vi "Dialog_Pause.vi"(11 "Wait (s)":dbl) -> ()   [LabVIEW 2012]
panel:
  in  "Cancel Button":bool
  out "Gauge":dbl(knob) scale=0.0..3.0
  out "Slide":dbl(slide) scale=0.0..3.0
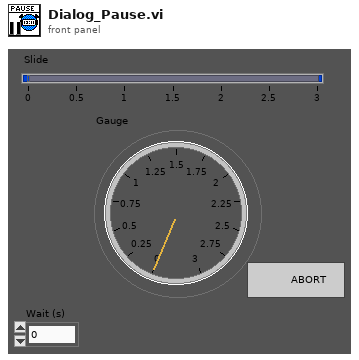
[diagram p1: front panel]
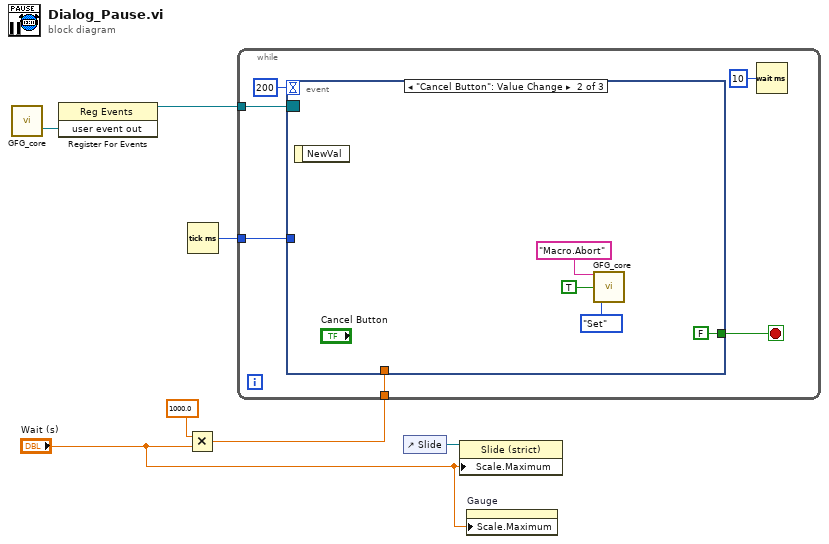
[diagram p0: block diagram]
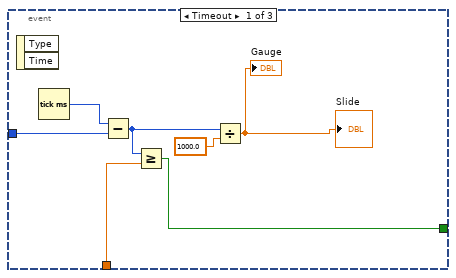
[diagram p2: hidden frame]
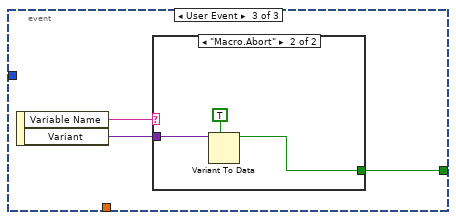
[diagram p3: hidden frame]
diagram:
  n1 = call "GFG_core.vi"() -> ("user event out"=w2:refnum<user-event>)  [unwired: 13 in, 6 out]
  n2 = register-events(w2) -> (reference out=w1:refnum<event-registration>)  [unwired: 2 in, 1 out]
  n3 = Multiply(x=1000.0 ("y"), y="Wait (s)") -> (x*y=w5:dbl)
  n4 = Tick Count (ms)() -> (millisecond timer value=w7:u32)
  n5 = while {
    tunnel: w5 -> [w13]
    tunnel: w7 -> [w12]
    tunnel: w1 -> [w8]
    stop <- w11 stop-if-true
    n6 = event shown="[1] \"Cancel Button\": Value Change" {
      selector: w8 -> [_ _ _]
      dyn-events: _ -> [_ _ _]
      timeout: 200 -> [_ _ _]
      tunnel: w13 -> [w19 _ _]
      tunnel: w12 -> [w16 _ _]
      tunnel: [w14 FALSE w26] -> w11
      event Timeout {
        n7 = event-data() -> ()  [unwired: 1 in, 2 out]
        n8 = Tick Count (ms)() -> (millisecond timer value=w20:u32)
        n9 = Subtract(x=w20, y=w16) -> (x-y=w17:u32)
        n10 = Greater Or Equal?(x=w17, y=w19) -> (x >= y?=w14:bool)
        n11 = Divide(x=w17, y=1000.0) -> (x/y=→"Slide" →"Gauge":dbl)
      }
      event "Cancel Button": Value Change {
        n12 = event-data() -> ()  [unwired: 1 in, 1 out]
        n13 = call "GFG_core.vi"("Variable Name in"="Macro.Abort", "Variant in"=TRUE, "Action"=enum16{"Init", "Set", "Get", "Clear"}."Set") -> ()  [unwired: 10 in, 7 out]
      }
      event User Event {
        n14 = event-data() -> ("Variable Name"=w27:string, "Variant"=w25:variant)  [unwired: 1 in]
        n15 = case shown="\"Macro.Abort\"" w27 {
          tunnel: [_ w28] -> w26
          tunnel: w25 -> [_ w30]
          frame Default {
          }
          frame "Macro.Abort" {
            n16 = Variant To Data(type=TRUE, Variant=w30) -> (data=w28:bool)  [unwired: 1 in, 1 out]
          }
        }
      }
    }
    n17 = Wait (ms)(milliseconds to wait=u32 10) -> ()  [unwired: 1 out]
  }
  n18 = control-ref of="Slide"() -> (w3:refnum<vi>)
  n19 = property on="Property Node" class="Slide (strict)"(reference=w3, "Scale.Maximum"="Wait (s)") -> ()  [unwired: 1 in, 2 out]
  n20 = property on="Gauge" class="Knob (strict)"("Scale.Maximum"="Wait (s)") -> ()  [unwired: 2 in, 2 out]
